vi "SetVelocitySetpoint.vi"(8 "xAxisSpeed":dbl, 9 "leftVelocitySetpointInput":dbl, 10 "rightVelocitySetpointInput":dbl, 11 "DriveBase.lvclass":refnum<class "DriveBase.lvclass">) -> (3 "DriveBase.lvclass 2":refnum<class "DriveBase.lvclass">)   [LabVIEW 2016, in "DriveBase.lvclass"]
uses:
  DriveBase.lvclass
  DriveBase.lvclass/DriveBase.ctl
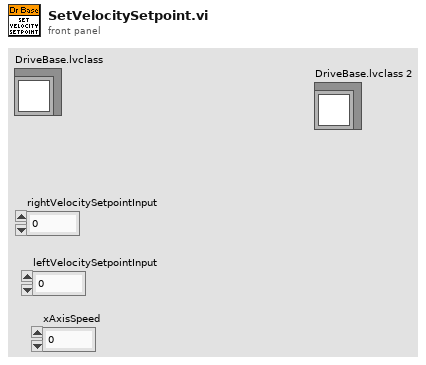
[diagram p1: front panel]
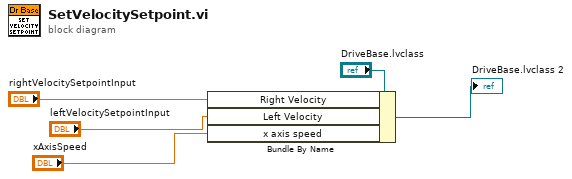
[diagram p0: block diagram]
diagram:
  n1 = Bundle By Name(cluster="DriveBase.lvclass", "Right Velocity"="rightVelocitySetpointInput", "Left Velocity"="leftVelocitySetpointInput", "x axis speed"="xAxisSpeed") -> (→"DriveBase.lvclass 2":refnum<class "DriveBase.lvclass">)
